vi "RunAbout_visible.vi"(11 "This VI":refnum<vi>) -> ()   [LabVIEW 2021]
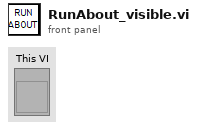
[diagram p1: front panel]
types:
  T1 = enum32{"invalid app kind", "Development System", "Run Time System", "Student Edition", "Embedded LabVIEW", "Evaluation", "Custom"}
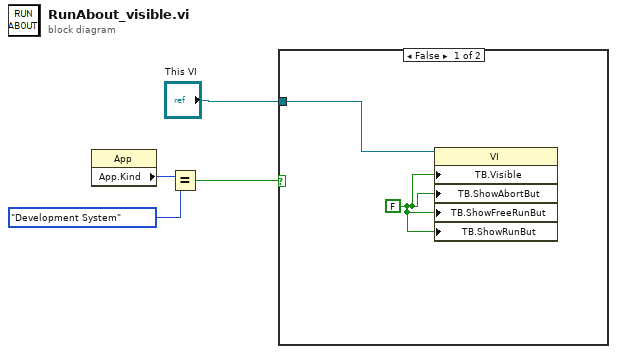
[diagram p0: block diagram]
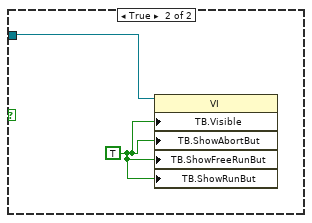
[diagram p2: hidden frame]
diagram:
  n1 = property class="App"() -> ("App.Kind"=w3:T1)  [unwired: 2 in, 2 out]
  n2 = Equal?(x=w3, y=T1."Development System") -> (x = y?=w2:bool)
  n3 = case shown="False" w2 {
    tunnel: "This VI" -> [w5 w7]
    frame False {
      w6 = FALSE ("Tool Bar:Visible")
      n4 = property class="VI"(reference=w5, "TB.Visible"=w6, "TB.ShowAbortBut"=w6, "TB.ShowFreeRunBut"=w6, "TB.ShowRunBut"=w6) -> ()  [unwired: 1 in, 2 out]
    }
    frame True {
      w8 = TRUE ("Tool Bar:Visible")
      n5 = property class="VI"(reference=w7, "TB.Visible"=w8, "TB.ShowAbortBut"=w8, "TB.ShowFreeRunBut"=w8, "TB.ShowRunBut"=w8) -> ()  [unwired: 1 in, 2 out]
    }
  }
